vi "Serialize.vi"(8 "error in (no error)":errorcluster, 10 "Element in":refnum<k20>, 11 "Property in":refnum<class "Property.lvclass">) -> (0 "error out":errorcluster, 2 "Element out":refnum<k20>)   [LabVIEW 2013, in "JUnit XML.lvlib" / "Property.lvclass"]
doc: "Serializes a Property using NI XML Parser."
uses:
  Property.lvclass
  Property.lvclass/Property.ctl
  <vilib>/xml/Close Reference(Node).vi
  <vilib>/xml/NI_XML.lvlib
  JUnit XML.lvlib
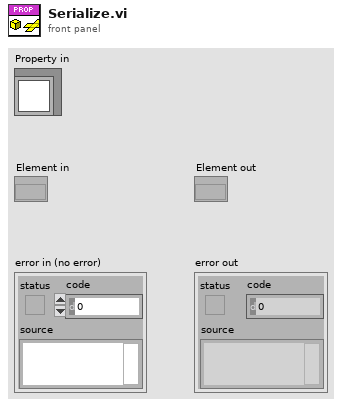
[diagram p1: front panel]
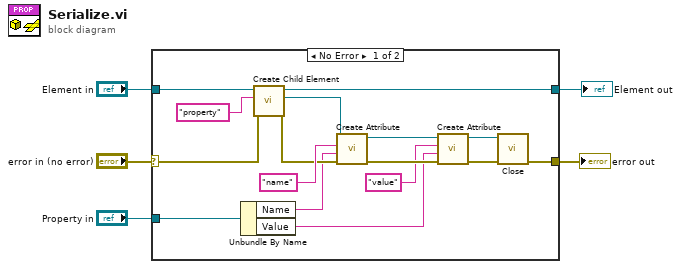
[diagram p0: block diagram]
diagram:
  n1 = case shown="No Error" "error in (no error)" {
    selector: "error in (no error)" -> [w10 w23]
    tunnel: [w9 w23] -> w4
    tunnel: "Property in" -> [w8 _]
    tunnel: "Element in" -> [w12 w22]
    tunnel: [w11 w22] -> w1
    frame No Error {
      n2 = Unbundle By Name(w8) -> ("Name"=w7:string, "Value"=w6:string)
      n3 = call "Create Child Element.vi"("error in (no error)"=w10, "Name"="property" ("Tag Name"), "Element in"=w12) -> ("error out"=w15:errorcluster, "Child Element"=w16:refnum<k20>, "Element out"=w11:refnum<k20>)  [unwired: 6 in]
      n4 = call "Create Attribute.vi"("error in (no error)"=w15, "Value"=w7, "Name"="name" ("Attribute Name"), "Element in"=w16) -> ("error out"=w18:errorcluster, "Element out"=w19:refnum<k20>)  [unwired: 6 in]
      n5 = call "Create Attribute.vi"("error in (no error)"=w18, "Value"=w6, "Name"="value" ("Attribute Name"), "Element in"=w19) -> ("error out"=w13:errorcluster, "Element out"=w14:refnum<k20>)  [unwired: 6 in]
      n6 = call-poly <vilib>:"Close.vi"("error in (no error)"=w13, "node"=w14) -> ("error out"=w9:errorcluster)  [unwired: 7 in]
    }
    frame Error {
    }
  }
  "error out" <- w4
  "Element out" <- w1
